vi "Main.vi"() -> ()   [LabVIEW 2014, in "Character Encoding Conversion.lvlib"]
doc: "Copyright (c) 2016 Sze Howe Koh\nThis code is licensed under the MIT license"
uses:
  Character Encoding Conversion.lvlib
  src/LabVIEW/LQ Core/LQIdentity/LQIdentity.lvclass/LQIdentity.ctl
  src/LabVIEW/Qt Widgets/QWidget/setWindowTitle.vi
  src/LabVIEW/Qt Widgets/QWidget/setFont.vi
  src/LabVIEW/Qt Widgets/QTextEdit/setReadOnly.vi
  src/LabVIEW/Qt Widgets/QWidget/setVisible.vi
  src/LabVIEW/LQ Core/LQCoreEngine/LQCoreEngine.lvclass
  src/LabVIEW/LQ Core/QTextCodec/QTextCodec.lvclass
  src/LabVIEW/Qt Widgets/QTextEdit/QTextEdit.lvclass
  src/LabVIEW/Qt GUI/QFont/QFont.lvclass
  src/LabVIEW/LQ Core/LQIdentity/LQIdentity.lvclass
panel:
  in  "Codec":string(combo)
  out "Decoded Byte Count":i32
  out "Input Byte Count":i32
  in  "Input Text File":path
  in  "Decode Button":bool
  in  "Stop Button":bool
  # "Prerequisite knowledge/experience\n- One of the \"Hello World\" examples\n\n- Character encoding\n   https://en.wikipedia.org/wiki/Character_encoding\n\n\nDescription\nBy default, LabVIEW assumes that all textual data is encoded according to your system locale. As a result, for\nexample, a Japanese version of LabVIEW cannot properly display Thai text. In contrast, LQ Widgets assumes\nthat all textual data is encoded in UTF-8, which supports the most of the languages in use today.\n\nYou can use a text codec to convert text from a non-local encoding to UTF-8, and vice-versa.\n\n\nInstructions\n1. Run this VI\n2. In the \"Input Text File\" field, select a file from the \"Resources\" folder of this example\n3. Select the Codec that matches your selected file\n4. Click \"Decode!\" and watch the \"Decoded Text\" window\n\n\nShowcase\n- Ability to parse text from a variety of encodings."
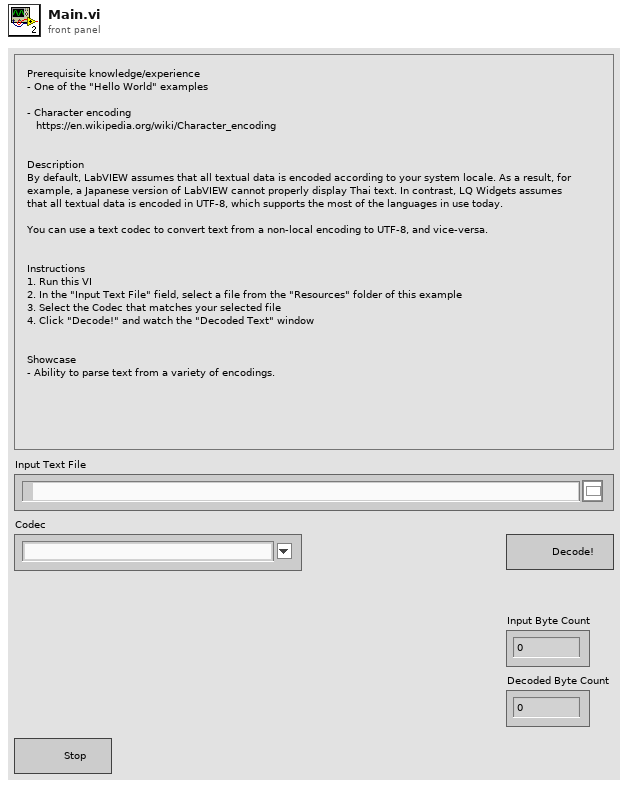
[diagram p1: front panel]
types:
  T1 = typedef "LVComboBoxStrsAndValuesArrayTypeDef.ctl" = cluster{"String":string, "Value":string}[]
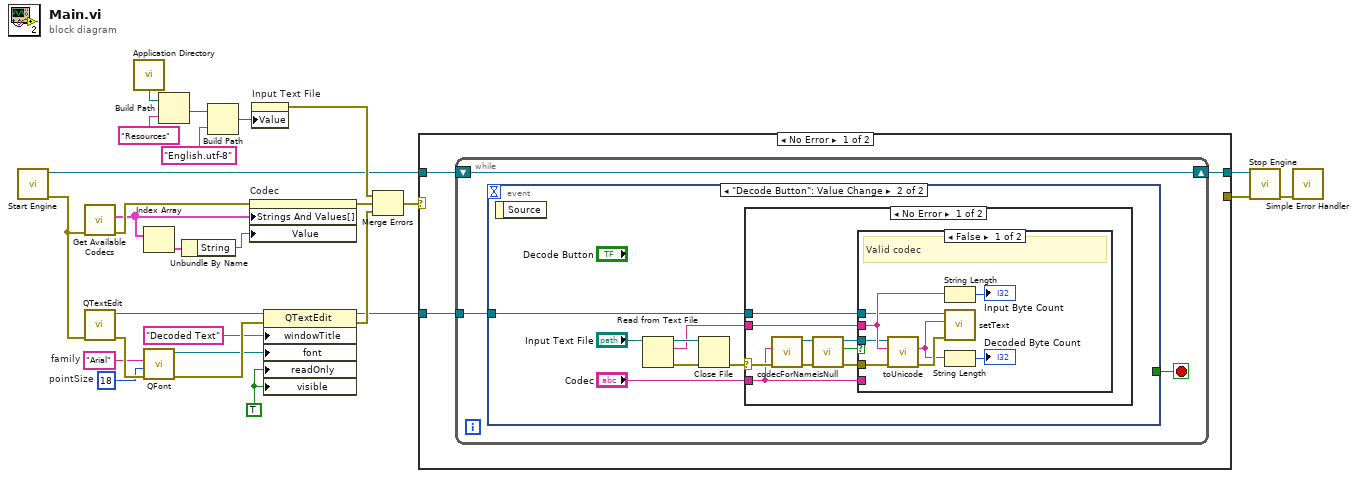
[diagram p0: block diagram]
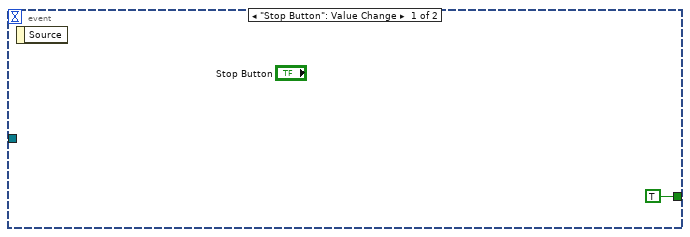
[diagram p2: hidden frame]
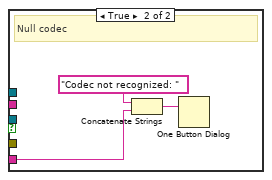
[diagram p3: hidden frame]
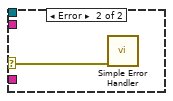
[diagram p4: hidden frame]
diagram:
  w16 = 18  # pointSize
  w17 = "Arial"  # family
  w14 = TRUE ("visible")
  n1 = call "Start Engine.vi"() -> ("Error Out"=w13:errorcluster, "New Engine"=w21:refnum<class "LQCoreEngine.lvclass">)  [unwired: 10 in]
  n2 = call "Get Available Codecs.vi"("Error In"=w13) -> ("Error Out"=w23:errorcluster, "Combo Box Items"=w10:T1)  [unwired: 9 in]
  n3 = call "QTextEdit.vi"("Error In"=w13) -> ("Error Out"=w26:errorcluster, "New QTextEdit"=w22:refnum<class "QTextEdit.lvclass">)  [unwired: 9 in]
  n4 = call <vilib>:"Application Directory.vi"() -> ("Application Directory"=w5:path)
  n5 = Index Array(array=w10) -> (element=w9:cluster{"String":string, "Value":string})  [unwired: 1 in]
  n6 = call "QFont.vi"("Error In"=w26, "pointSize"=w16, "family"=w17) -> ("Error Out"=w25:errorcluster, "New QFont"=w15:refnum<class "QFont.lvclass">)  [unwired: 7 in]
  n7 = Build Path(base path=w5, name or relative path="Resources") -> (appended path=w3:path)
  n8 = Unbundle By Name(w9) -> ("String"=w8:string)
  n9 = Build Path(base path=w3, name or relative path="English.utf-8") -> (appended path=w1:path)
  n10 = property on="Codec" class="CmbBox"(error in=w23, "Strings And Values[]"=w10, "Value"=w8) -> (error out=w12:errorcluster)  [unwired: 1 in, 1 out]
  n11 = property on="Input Text File" class="Path"("Value"=w1) -> (error out=w27:errorcluster)  [unwired: 2 in, 1 out]
  n12 = property class="QTextEdit"(reference=w22, error in=w25, "windowTitle"="Decoded Text", "font"=w15, "readOnly"=w14, "visible"=w14) -> (reference out=w19:refnum<class "QTextEdit.lvclass">, error out=w24:errorcluster)
  n13 = Merge Errors(w27, w12, w24) -> (w11:errorcluster)
  n14 = case shown="No Error" w11 {
    selector: w11 -> [_ w62]
    tunnel: w21 -> [w30 w63]
    tunnel: [w29 w63] -> w20
    tunnel: w19 -> [w28 _]
    tunnel: [_ w62] -> w7
    frame No Error {
      n15 = while {
        shift-right: [w32] -> w29
        shift-left: w30 -> [w32]
        tunnel: w28 -> [w31]
        stop <- w33 stop-if-true
        n16 = event shown="[1] \"Decode Button\": Value Change" {
          selector: _ -> [_ _]
          dyn-events: _ -> [_ _]
          timeout: _ -> [_ _]
          tunnel: [TRUE _] -> w33
          tunnel: w31 -> [_ w36]
          event "Stop Button": Value Change {
            n17 = event-data() -> ()  [unwired: 1 in, 1 out]
          }
          event "Decode Button": Value Change {
            n18 = event-data() -> ()  [unwired: 1 in, 1 out]
            n19 = Read from Text File(file (use dialog)="Input Text File") -> (refnum out=w39:refnum<file>, text=w38:string, error out=w41:errorcluster)  [unwired: 3 in, 1 out]
            n20 = Close File(refnum=w39, error in=w41) -> (error out=w37:errorcluster)  [unwired: 1 out]
            n21 = case shown="No Error" w37 {
              selector: w37 -> [w47 w61]
              tunnel: "Codec" -> [w42 _]
              tunnel: w38 -> [w49 _]
              tunnel: w36 -> [w46 _]
              frame No Error {
                n22 = call "codecForName.vi"("Error In"=w47, "name"=w42) -> ("Error Out"=w48:errorcluster, "New QTextCodec"=w45:refnum<class "QTextCodec.lvclass">)  [unwired: 8 in]
                n23 = call "isNull.vi"("LQIdentity In"=w45) -> ("Is Null?"=w43:bool, "LQIdentity Out"=w44:refnum<class "QTextCodec.lvclass">)  [unwired: 9 in]
                n24 = case shown="False" w43 {
                  tunnel: w49 -> [w56 _]
                  tunnel: w48 -> [w53 _]
                  tunnel: w46 -> [w52 _]
                  tunnel: w44 -> [w50 _]
                  tunnel: w42 -> [_ w59]
                  frame False {
                    # "Valid codec"
                    n25 = call "toUnicode.vi"("Error In"=w53, "string"=w56, "QTextCodec In"=w50) -> ("Error Out"=w57:errorcluster, "Value"=w51:string)  [unwired: 6 in, 1 out]
                    n26 = String Length(string=w56) -> (length=→"Input Byte Count":i32)
                    n27 = call "setText.vi"("Error In"=w57, "text"=w51, "QTextEdit In"=w52) -> ()  [unwired: 7 in, 2 out]
                    n28 = String Length(string=w51) -> (length=→"Decoded Byte Count":i32)
                  }
                  frame True {
                    # "Null codec"
                    n29 = Concatenate Strings("Codec not recognized: " ("string"), w59) -> (w58:string)
                    n30 = One Button Dialog(message=w58) -> ()  [unwired: 1 in, 1 out]
                  }
                }
              }
              frame Error {
                n31 = call <vilib>:"Simple Error Handler.vi"("error in (no error)"=w61) -> ()  [unwired: 4 in, 5 out]
              }
            }
          }
        }
      }
    }
    frame Error {
    }
  }
  n32 = call "Stop Engine.vi"("Error In"=w7, "LQCoreEngine"=w20) -> ("Error Out"=w6:errorcluster)  [unwired: 9 in]
  n33 = call <vilib>:"Simple Error Handler.vi"("error in (no error)"=w6) -> ()  [unwired: 4 in, 5 out]
